vi "NotifyUIState.vi"(8 "error in (no error)":errorcluster, 10 "UI State":T1, 11 "Home":refnum<class "Home.lvclass">) -> (0 "error out":errorcluster, 3 "Home out":refnum<class "Home.lvclass">)   [LabVIEW 2022 SP3, in "Home.lvclass"]
uses:
  Home.lvclass
  Home.lvclass/Home.ctl
  Typedefs/Home State--enum.ctl
panel:
  # "For instructions on how to use the JKI State Machine Objects, examples and video tutorials, visit:\nhttp://jki.net/state-machine-objects/\n\nJKI State Machine Objects™\nhttp://jki.net/state-machine-objects/\nCopyright (C) 2005-2015, JKI <info@jki.net>\nALL RIGHTS RESERVED"
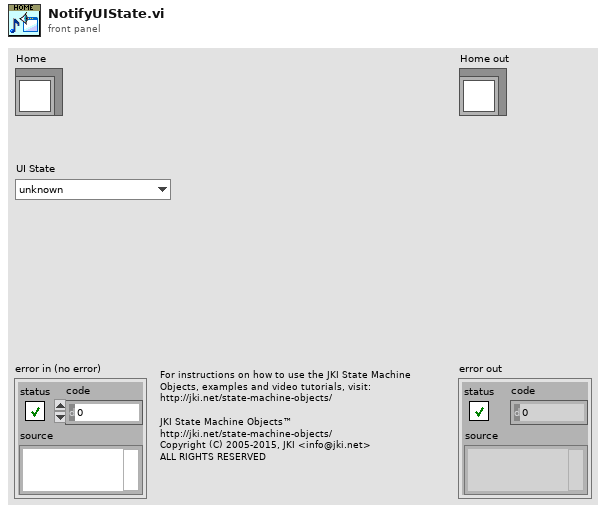
[diagram p1: front panel]
types:
  T1 = typedef "Home.lvclass/Home State--enum.ctl" = enum16{"unknown", "Opened", "Embedded", "Closed"}
  T2 = typedef "Home.lvclass/PublicEvents--Cluster.ctl" = cluster{"UI State":refnum<user-event>}
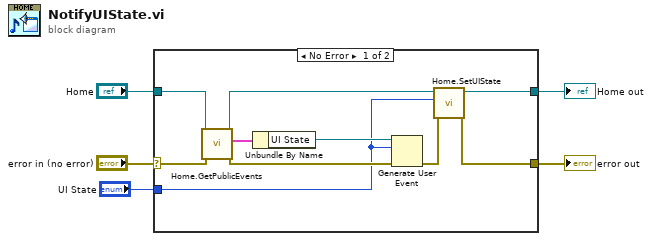
[diagram p0: block diagram]
diagram:
  n1 = case shown="No Error" "error in (no error)" {
    selector: "error in (no error)" -> [w14 w17]
    tunnel: [w6 w17] -> w4
    tunnel: [w9 w16] -> w2
    tunnel: "Home" -> [w15 w16]
    tunnel: "UI State" -> [w8 _]
    frame No Error {
      n2 = call "Home.GetPublicEvents.vi"("error in (no error)"=w14, "Home"=w15) -> ("error out"=w11:errorcluster, "SMO.UI Public Events"=w13:T2, "Home out"=w10:refnum<class "Home.lvclass">)  [unwired: 7 in]
      n3 = Unbundle By Name(w13) -> ("UI State"=w12:refnum<user-event>)
      n4 = Generate User Event(user event=w12, event data cluster=w8, error in=w11) -> (error out=w7:errorcluster)  [unwired: 1 in, 1 out]
      n5 = call "Home.SetUIState.vi"("error in (no error)"=w7, "UI State"=w8, "Home"=w10) -> ("error out"=w6:errorcluster, "Home out"=w9:refnum<class "Home.lvclass">)  [unwired: 7 in]
    }
    frame Error {
    }
  }
  "error out" <- w4
  "Home out" <- w2
